vi "Make Receiver.vi"(8 "error in (no error)":errorcluster, 11 "Concrete Message Rescripter in":refnum<class "Concrete Message Rescripter.lvclass">) -> (0 "error out":errorcluster, 3 "Concrete Message Rescripter out":refnum<class "Concrete Message Rescripter.lvclass">)   [LabVIEW 2020, in "Message Rescripter.lvlib" / "Concrete Message Rescripter.lvclass"]
uses:
  Concrete Message Rescripter.lvclass
  MessageMakerProvider/_Message Maker/_Maker Classes/Concrete Message Scripter/Concrete Message Scripter.lvclass
  MessageMakerProvider/_Message Maker/_Maker Classes/Message Scripter/Message Scripter.lvclass
  Message Rescripter.lvlib
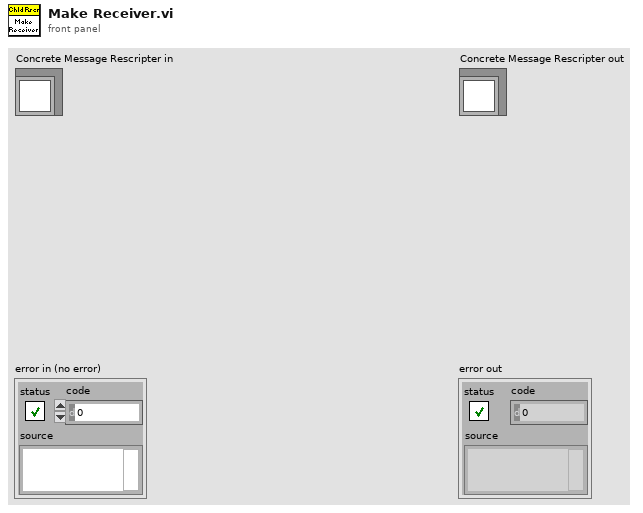
[diagram p1: front panel]
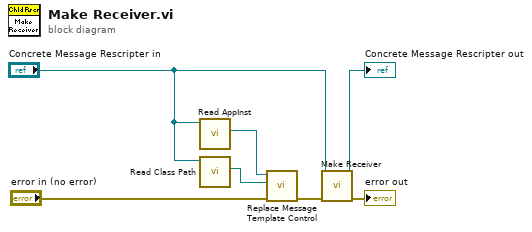
[diagram p0: block diagram]
diagram:
  n1 = call "Read AppInst.vi"("Message Maker in"="Concrete Message Rescripter in") -> ("AppInst"=w5:refnum<vi>)  [unwired: 10 in]
  n2 = call "Read Class Path.vi"("Message Scripter in"="Concrete Message Rescripter in") -> ("Class Path"=w4:path)  [unwired: 10 in]
  n3 = call "Replace Message Template Control.vi"("error in (no error)"="error in (no error)", "Class Path"=w4, "App Inst"=w5) -> ("error out"=w2:errorcluster)  [unwired: 8 in]
  n4 = call-parent "Make Receiver.vi"("error in (no error)"=w2, "Concrete Message Scripter in"="Concrete Message Rescripter in") -> ("error out"=→"error out":errorcluster, "Concrete Message Scripter out"=→"Concrete Message Rescripter out":refnum<class "Concrete Message Rescripter.lvclass">)  [unwired: 8 in]
